vi "bindata descr by kwarg_name.vi"(8 "Error in":errorcluster, 9 "kwarg_name":string, 11 "Bindata & descr":T1) -> (0 "Error out":errorcluster, 1 "index":i32, 2 "bindata descr":T2={"nofbytes"=0, "numtype"="", "start"=0, "arrdims"=[], "kwarg_name"="", "category"="numarrays"}, 3 "Bindata & descr out":T1)   [LabVIEW 2018, in "LV2Julia_core.lvlib"]
uses:
  LV2Julia_core.lvlib
  Bindata description.ctl
  Bindata&description.ctl
  <vilib>/Utility/error.llb/Error Cluster From Error Code.vi
  <vilib>/ErrorRing/Error Ring.xnode
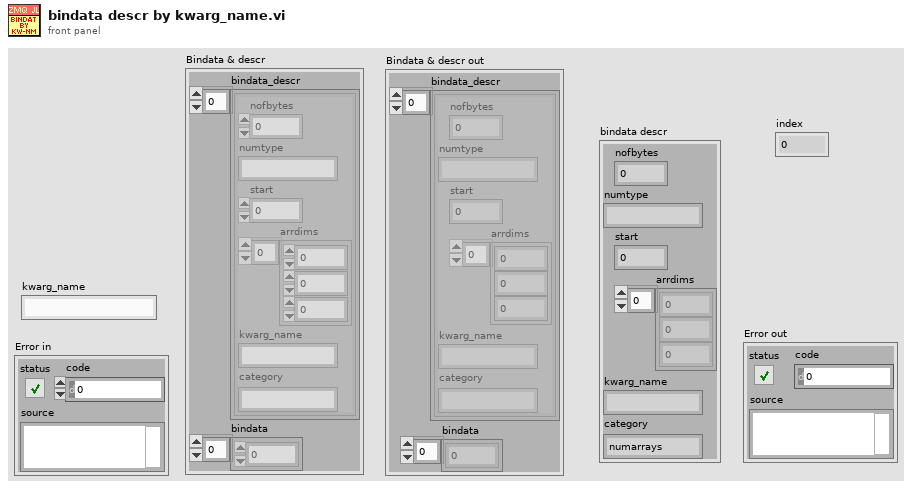
[diagram p1: front panel]
types:
  T1 = typedef "LV2Julia_core.lvlib/Bindata&description.ctl" = cluster{"bindata_descr":T2[], "bindata":u8[]}
  T2 = typedef "LV2Julia_core.lvlib/Bindata description.ctl" = cluster{"nofbytes":i32, "numtype":string, "start":i32, "arrdims":i32[], "kwarg_name":string, "category":string}
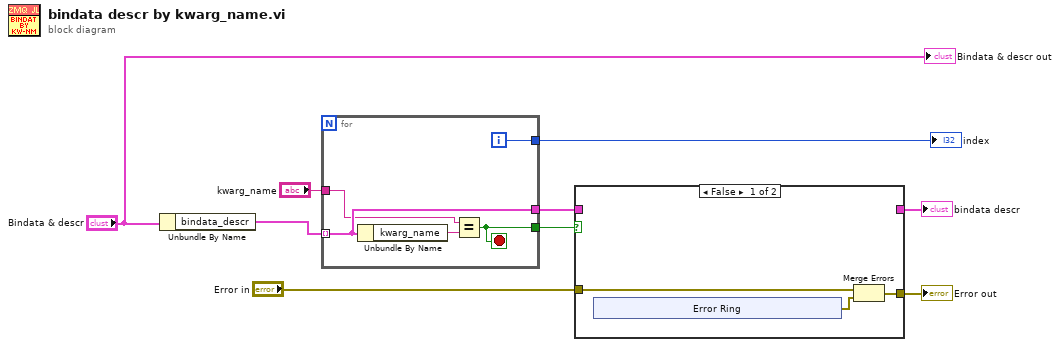
[diagram p0: block diagram]
diagram:
  n1 = Unbundle By Name("Bindata & descr") -> ("bindata_descr"=w1:T2[])
  n2 = for {
    tunnel: w1 -> [w14] mode=indexing
    tunnel: [w14] -> w5
    tunnel: "kwarg_name" -> [w12]
    tunnel: [w11] -> w4
    tunnel: [w10] -> w3
    i -> [w10]
    stop <- w11 stop-if-true
    n3 = Unbundle By Name(w14) -> ("kwarg_name"=w13:string)
    n4 = Equal?(x=w12, y=w13) -> (x = y?=w11:bool)
  }
  "index" <- w3
  n5 = case shown="False" w4 {
    tunnel: [_ w23] -> w7
    tunnel: w5 -> [_ w23]
    tunnel: [w16 w22] -> w6
    tunnel: "Error in" -> [w17 w22]
    frame False {
      n6 = xnode "Error Ring"() -> ("error out"=w15:errorcluster)
      n7 = Merge Errors(w17, w15) -> (w16:errorcluster)
    }
    frame True {
    }
  }
  "bindata descr" <- w7
  "Error out" <- w6
  "Bindata & descr out" <- "Bindata & descr"
